vi "初始化 1.vi"(3 "Container State":T4 caption="容器状态", 4 "Previous State":variant caption="前期状态", 5 "Previous Version":T3 caption="前期版本") -> (2 "Current State":T1={"模块启用"={"原位多参数"=FALSE, "集成式多参数"=FALSE, "营养盐"=FALSE}, "模块名称"={"原位多参数"="环境动力", "集成式多参数"="氨氮", "营养盐"="总磷"}} caption="当前状态")   [LabVIEW 2016, in "运维调试菜单.xctl"]
uses:
  <vilib>/_xctls/Container State.ctl
  <vilib>/_xctls/Version.ctl
  <vilib>/_xctls/XControlSupport.lvlib
panel:
  in  "State 2":T1={"模块启用"={"原位多参数"=FALSE, "集成式多参数"=FALSE, "营养盐"=FALSE}, "模块名称"={"原位多参数"="环境动力", "集成式多参数"="氨氮", "营养盐"="总磷"}} caption="状态"
  in  "State":T1={"模块启用"={"原位多参数"=TRUE, "集成式多参数"=TRUE, "营养盐"=TRUE}, "模块名称"={"原位多参数"="原位多参数", "集成式多参数"="集成多参数", "营养盐"="营养盐"}} caption="默认输入控件状态"
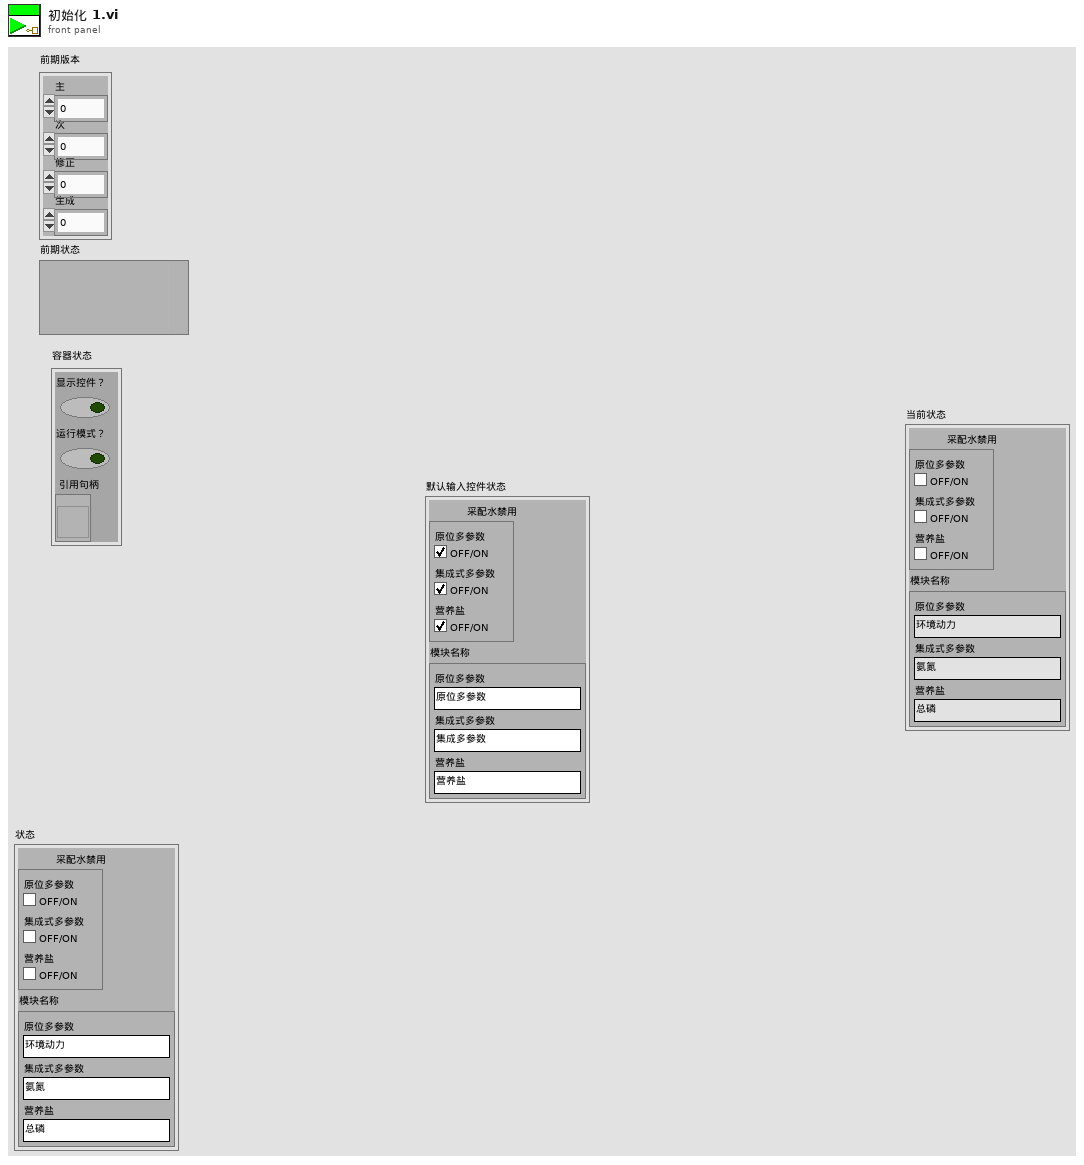
[diagram p1: front panel]
types:
  T1 = typedef "运维调试菜单.xctl/状态 1.ctl" = cluster{"模块启用":T2, "模块名称":cluster{"原位多参数":string, "集成式多参数":string, "营养盐":string}}
  T2 = typedef "运维调试菜单.xctl/模块启用.ctl" = cluster{"原位多参数":bool, "集成式多参数":bool, "营养盐":bool}
  T3 = typedef "XControlSupport.lvlib/Version.ctl" = cluster{"Major":u16, "Minor":u16, "Fix":u16, "Build":u16}
  T4 = typedef "XControlSupport.lvlib/Container State.ctl" = cluster{"Indicator?":bool, "Run Mode?":bool, " Refnum":refnum<vi>}
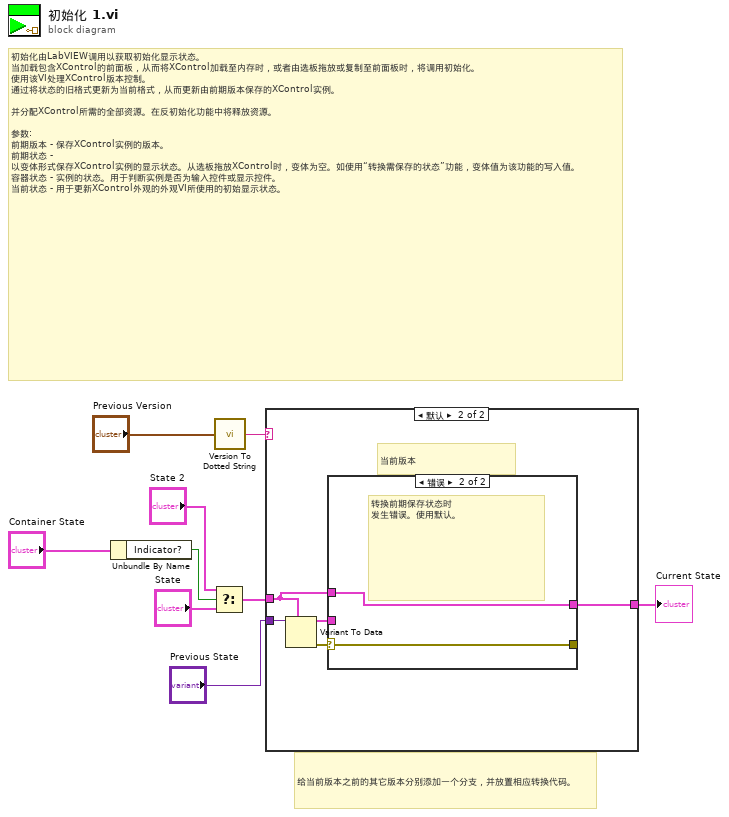
[diagram p0: block diagram]
diagram:
  # "给当前版本之前的其它版本分别添加一个分支，并放置相应转换代码。"
  # "初始化由LabVIEW调用以获取初始化显示状态。\n当加载包含XControl的前面板，从而将XControl加载至内存时，或者由选板拖放或复制至前面板时，将调用初始化。\n使用该VI处理XControl版本控制。\n通过将状态的旧格式更新为当前格式，从而更新由前期版本保存的XControl实例。\n\n并分配XControl所需的全部资源。在反初始化功能中将释放资源。\n\n参数: \n前期版本 - 保存XControl实例的版本。\n前期状态 - 以变体形式保存XControl实例的显示状态。从选板拖放XControl时，变体为空。如使用“转换需保存的状态”功能，变体值为该功能的写入值。\n容器状态 - 实例的状态。用于判断实例是否为输入控件或显示控件。\n当前状态 - 用于更新XControl外观的外观VI所使用的初始显示状态。"
  n1 = Unbundle By Name("Container State") -> ("Indicator?"=w7:bool)
  n2 = Select(t="State 2", s=w7, f="State") -> (s? t:f=w6:T1)
  n3 = call <vilib>:"Version To Dotted String.vi"("Version"="Previous Version") -> ("String Version"=w4:string)
  n4 = case shown="默认" w4 {
    tunnel: "Previous State" -> [_ w15]
    tunnel: [w10 w11] -> w1
    tunnel: w6 -> [w10 w12]
    frame "0.0.0.0" {
      # "已创建，并使用默认状态"
    }
    frame Default {
      # "当前版本"
      n5 = Variant To Data(type=w12, Variant=w15) -> (data=w13:T1, error out=w14:errorcluster)  [unwired: 1 in]
      n6 = case shown="错误" w14 {
        selector: w14 -> [w17 w18]
        tunnel: w13 -> [w16 _]
        tunnel: [w16 w19] -> w11
        tunnel: w12 -> [_ w19]
        tunnel: [w17 w18] -> _
        frame No Error {
        }
        frame Error {
          # "转换前期保存状态时\n发生错误。使用默认。"
        }
      }
    }
  }
  "Current State" <- w1
